vi "BuildLinString.vi"(0 "X0":dbl, 1 "Y0":dbl, 2 "X0 graph pixels":i32, 3 "Y0 graph pixels":i32, 5 "X1":dbl, 11 "error in (no error)":errorcluster, 12 "Y1":dbl, 13 "X1 graph pixels":i32, 14 "Y1 graph pixels":i32) -> (4 "String":string, 15 "error out":errorcluster)   [LabVIEW 2023]
doc: "Builds a line string from format globals and points values."
uses:
  StringFormatGlobals.vi
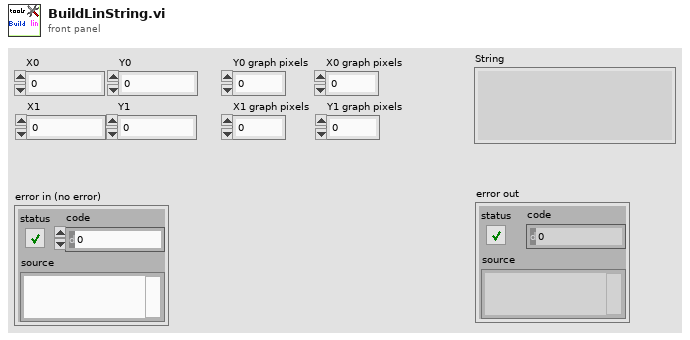
[diagram p1: front panel]
types:
  T1 = typedef "LinFormatString.ctl" = string
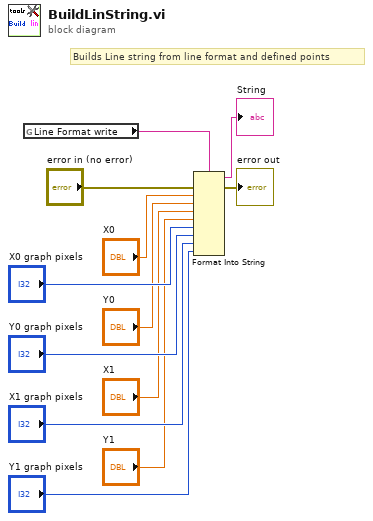
[diagram p0: block diagram]
diagram:
  # "Builds Line string from line format and defined points"
  n1 = global read "StringFormatGlobals.vi" "Line Format write"() -> (w8:T1)
  n2 = Format Into String(format string=w8, error in="error in (no error)", "X0", "Y0", "X1", "Y1", "X0 graph pixels", "Y0 graph pixels", "X1 graph pixels", "Y1 graph pixels") -> (resulting string=→"String":string, error out=→"error out":errorcluster)  [unwired: 1 in]
